vi "HFRR ADV v04.vi"() -> ()   [LabVIEW 2025] (continued)
                }
                frame 94 {
                  n2376 = local write "S 96"(w3499) -> ()
                }
                frame 95 {
                  n2377 = local write "S 97"(w3500) -> ()
                }
                frame 96 {
                  n2378 = local write "S 98"(w3501) -> ()
                }
                frame 97 {
                  n2379 = local write "S 99"(w3502) -> ()
                }
                frame 98 {
                  n2380 = local write "S 100"(w3503) -> ()
                }
                frame 99 {
                  n2381 = local write "S 101"(w3504) -> ()
                }
                frame 100 {
                  n2382 = local write "S 102"(w3505) -> ()
                }
                frame 101 {
                  n2383 = local write "S 103"(w3506) -> ()
                }
                frame 102 {
                  n2384 = local write "S 104"(w3507) -> ()
                }
                frame 103 {
                  n2385 = local write "S 105"(w3508) -> ()
                }
                frame 104 {
                  n2386 = local write "S 106"(w3509) -> ()
                }
                frame 105 {
                }
                frame 106 {
                  n2387 = property on="OK Button 17" class="Bool (strict)"("Boolean Text.Text"=w3510) -> ()  [unwired: 2 in, 2 out]
                }
                frame 107 {
                  n2388 = property on="OK Button 16" class="Bool (strict)"("Boolean Text.Text"=w3511) -> ()  [unwired: 2 in, 2 out]
                }
                frame 108 {
                  n2389 = property on="TITTLE" class="Str"("Caption.Text"=w3512) -> ()  [unwired: 2 in, 2 out]
                }
                frame 109 {
                  "String 30" <- w3513
                }
                frame 110 {
                  n2390 = property on="Test Date" class="Str"("Caption.Text"=w3514) -> ()  [unwired: 2 in, 2 out]
                  "String 31" <- w3514
                }
                frame 111 {
                  n2391 = property on="Sample ID" class="Str"("Caption.Text"=w3515) -> ()  [unwired: 2 in, 2 out]
                  "String 32" <- w3515
                }
                frame 112 {
                  n2392 = property on="Tested by" class="Str"("Caption.Text"=w3516) -> ()  [unwired: 2 in, 2 out]
                  "String 33" <- w3516
                }
                frame 113 {
                  n2393 = property on="System Configured Printers 2" class="Arr (strict)"("Caption.Text"=w3517) -> ()  [unwired: 2 in, 2 out]
                }
                frame 114 {
                  n2394 = property on="Selected Printer" class="Str"("Caption.Text"=w3518) -> ()  [unwired: 2 in, 2 out]
                }
                frame 115 {
                  n2395 = property on="Select Printer 3" class="DigNum (strict)"("Caption.Text"=w3519) -> ()  [unwired: 2 in, 2 out]
                }
                frame 116 {
                  n2396 = property on="Print" class="Bool (strict)"("Boolean Text.Text"=w3520) -> ()  [unwired: 2 in, 2 out]
                }
                frame 117 {
                  "String 41" <- w3521
                }
                frame 118 {
                  n2397 = property on="tested by" class="Str"("Caption.Text"=w3522) -> ()  [unwired: 2 in, 2 out]
                }
                frame 119 {
                }
                frame 120 {
                  n2398 = property on="Export" class="Bool (strict)"("Boolean Text.Text"=w3523) -> ()  [unwired: 2 in, 2 out]
                }
                frame 121 {
                  n2399 = property on="TEMP INTERCEPT:" class="DigNum (strict)"("Caption.Text"=w3524) -> ()  [unwired: 2 in, 2 out]
                }
                frame 122 {
                  n2400 = property on="AIR TEMP INTERCEPT:" class="DigNum (strict)"("Caption.Text"=w3525) -> ()  [unwired: 2 in, 2 out]
                }
                frame 123 {
                  n2401 = property on="Select File Type" class="Enum (strict)"("Caption.Text"=w3526) -> ()  [unwired: 2 in, 2 out]
                }
                frame 124 {
                  n2402 = property on="s.NO" class="Str"("Caption.Text"=w3527) -> ()  [unwired: 2 in, 2 out]
                  "String 45" <- w3527
                }
                frame 125 {
                  n2403 = property on="trip1 8" class="Bool (strict)"("Boolean Text.Text"=w3528) -> ()  [unwired: 2 in, 2 out]
                }
                frame 126, Default {
                }
              }
            }
          }
          frame #1 {
            w3536 = TRUE ("Visible")
            n2404 = local read "S 91"() -> (w3553:string)
            n2405 = local read "S 90"() -> (w3552:string)
            n2406 = local read "S 88"() -> (w3551:string)
            n2407 = property on="Threshold" class="DigNum (strict)"("Caption.Text"=w3553) -> ()  [unwired: 2 in, 2 out]
            n2408 = property on="File Path" class="Path"("Caption.Text"=w3552) -> ()  [unwired: 2 in, 2 out]
            n2409 = property on="SrvM CP" class="Bool (strict)"("Boolean Text.Text"=w3551) -> ()  [unwired: 2 in, 2 out]
            n2410 = local read "S 71"() -> (w3546:string)
            n2411 = local read "S 86"() -> (w3548:string)
            n2412 = local read "S 85"() -> (w3549:string)
            n2413 = local read "S 87"() -> (w3547:string)
            n2414 = local read "S 84"() -> (w3550:string)
            n2415 = local read "S 103"() -> (w3535:string)
            n2416 = local read "S 104"() -> (w3534:string)
            n2417 = property on="ENTER THE NEW PASSWORD" class="Str"("Caption.Text"=w3547) -> ()  [unwired: 2 in, 2 out]
            n2418 = property on="Password" class="Str"("Caption.Text"=w3549) -> ()  [unwired: 2 in, 2 out]
            n2419 = property on="ENTER CURRENT PASSWORD" class="Str"("Caption.Text"=w3548) -> ()  [unwired: 2 in, 2 out]
            n2420 = property on="EDIT" class="Bool (strict)"("Boolean Text.Text"=w3546) -> ()  [unwired: 2 in, 2 out]
            n2421 = property on="SAVE" class="Bool (strict)"("Boolean Text.Text"=w3550) -> ()  [unwired: 2 in, 2 out]
            n2422 = Build Array(w3535, w3534) -> (w3533:string[])
            n2423 = property on="Heater Button" class="Bool (strict)"("Strings [4]"=w3533) -> ()  [unwired: 2 in, 2 out]
            n2424 = property on="CH-HUMIDITY WET" class="DigNum (strict)"("Caption.Size to Text?"=w3536) -> ()  [unwired: 2 in, 2 out]
            n2425 = property on="CH-HUMIDITY DRY" class="DigNum (strict)"("Caption.Size to Text?"=w3536) -> ()  [unwired: 2 in, 2 out]
            n2426 = property on="CH-POWER -" class="DigNum (strict)"("Caption.Size to Text?"=w3536) -> ()  [unwired: 2 in, 2 out]
            n2427 = property on="CH-HEATER" class="DigNum (strict)"("Caption.Size to Text?"=w3536) -> ()  [unwired: 2 in, 2 out]
            n2428 = property on="CH-POWER +" class="DigNum (strict)"("Caption.Size to Text?"=w3536) -> ()  [unwired: 2 in, 2 out]
            n2429 = local read "S 92"() -> (w3545:string)
            n2430 = local read "S 93"() -> (w3544:string)
            n2431 = local read "S 105"() -> (w3531:string)
            n2432 = local read "S 106"() -> (w3530:string)
            n2433 = Build Array(w3545, w3544) -> ()  [unwired: 1 out]
            n2434 = Build Array(w3531, w3530) -> (w3532:string[])
            n2435 = local read "S 95"() -> (w3542:string)
            n2436 = local read "S 94"() -> (w3543:string)
            n2437 = local read "bs"() -> (w3558:string)
            n2438 = local read "as"() -> (w3559:string)
            n2439 = property on="Humidity" class="Bool (strict)"("Strings [4]"=w3532) -> ()  [unwired: 2 in, 2 out]
            n2440 = Concatenate Strings(w3558, "\r", w3559) -> ()  [unwired: 1 out]
            n2441 = property on="STROKE GAIN :" class="DigNum (strict)"("Caption.Text"=w3542) -> ()  [unwired: 2 in, 2 out]
            n2442 = property on="DISPLACEMENT :" class="DigNum (strict)"("Caption.Text"=w3543) -> ()  [unwired: 2 in, 2 out]
            n2443 = property on="Rh After" class="DigNum (strict)"("Caption.Size to Text?"=TRUE ("Caption.Size to Text")) -> ()  [unwired: 2 in, 2 out]
            n2444 = local read "S 48"() -> (w3582:string)
            n2445 = local read "S 50"() -> (w3580:string)
            n2446 = local read "S 51"() -> (w3579:string)
            n2447 = local read "S 49"() -> (w3581:string)
            n2448 = local read "S 52"() -> (w3578:string)
            n2449 = local read "as"() -> (w3563:string)
            n2450 = local read "bs"() -> (w3564:string)
            n2451 = local read "S 56"() -> (w3577:string)
            n2452 = local read "S 57"() -> (w3576:string)
            n2453 = local read "S 58"() -> (w3575:string)
            n2454 = local read "S 59"() -> (w3574:string)
            n2455 = property on="OPEN" class="Bool (strict)"("Boolean Text.Text"=w3578) -> ()  [unwired: 2 in, 2 out]
            n2456 = property on="OPEN 1" class="Bool (strict)"("Boolean Text.Text"=w3582) -> ()  [unwired: 2 in, 2 out]
            n2457 = property on="OPEN 2" class="Bool (strict)"("Boolean Text.Text"=w3581) -> ()  [unwired: 2 in, 2 out]
            n2458 = property on="OPEN 3" class="Bool (strict)"("Boolean Text.Text"=w3580) -> ()  [unwired: 2 in, 2 out]
            n2459 = property on="OPEN 4" class="Bool (strict)"("Boolean Text.Text"=w3579) -> ()  [unwired: 2 in, 2 out]
            n2460 = Concatenate Strings(w3564, "\r", w3563) -> ()  [unwired: 1 out]
            n2461 = local read "S 102"() -> (w3537:string)
            n2462 = property on="КОФ1" class="DigNum (strict)"("Caption.Text"=w3577) -> ()  [unwired: 2 in, 2 out]
            n2463 = local read "S 98"() -> (w3541:string)
            n2464 = local read "S 99"() -> (w3540:string)
            n2465 = local read "S 100"() -> (w3539:string)
            n2466 = local read "S 101"() -> (w3538:string)
            n2467 = property on="КОФ2" class="DigNum (strict)"("Caption.Text"=w3576) -> ()  [unwired: 2 in, 2 out]
            n2468 = property on="КОФ3" class="DigNum (strict)"("Caption.Text"=w3575) -> ()  [unwired: 2 in, 2 out]
            n2469 = property on="КОФ4" class="DigNum (strict)"("Caption.Text"=w3574) -> ()  [unwired: 2 in, 2 out]
            n2470 = local read "bs"() -> (w3562:string)
            n2471 = local read "as"() -> (w3561:string)
            n2472 = property on="CH-POWER +" class="DigNum (strict)"("Caption.Text"=w3541) -> ()  [unwired: 2 in, 2 out]
            n2473 = property on="CH-POWER -" class="DigNum (strict)"("Caption.Text"=w3540) -> ()  [unwired: 2 in, 2 out]
            n2474 = property on="CH-HEATER" class="DigNum (strict)"("Caption.Text"=w3539) -> ()  [unwired: 2 in, 2 out]
            n2475 = property on="CH-HUMIDITY DRY" class="DigNum (strict)"("Caption.Text"=w3538) -> ()  [unwired: 2 in, 2 out]
            n2476 = property on="CH-HUMIDITY WET" class="DigNum (strict)"("Caption.Text"=w3537) -> ()  [unwired: 2 in, 2 out]
            n2477 = local read "S 60"() -> (w3573:string)
            n2478 = local read "S 54"() -> (w3583:string)
            n2479 = Concatenate Strings(w3562, "\r", w3561) -> ()  [unwired: 1 out]
            n2480 = Concatenate Strings(w3583, w3573) -> ()  [unwired: 1 out]
            n2481 = local read "S 77"() -> (→"String 43":string)
            n2482 = local read "S 76"() -> (w3556:string)
            n2483 = local read "S 78"() -> (w3555:string)
            n2484 = local read "S 71"() -> (w3567:string)
            n2485 = local read "S 66"() -> (w3572:string)
            n2486 = local read "S 67"() -> (w3571:string)
            n2487 = local read "S 68"() -> (w3570:string)
            n2488 = local read "S 69"() -> (w3569:string)
            n2489 = local read "S 70"() -> (w3568:string)
            n2490 = property on="AIR TEMP" class="DigNum (strict)"("Caption.Text"=w3555) -> ()  [unwired: 2 in, 2 out]
            n2491 = property on="Set Strk" class="DigNum (strict)"("Caption.Text"=w3556) -> ()  [unwired: 2 in, 2 out]
            n2492 = property on="FRIC. FORCE :" class="DigNum (strict)"("Caption.Text"=w3572) -> ()  [unwired: 2 in, 2 out]
            n2493 = property on="TEMPERATURE :" class="DigNum (strict)"("Caption.Text"=w3571) -> ()  [unwired: 2 in, 2 out]
            n2494 = property on="SPEED OUT:" class="DigNum (strict)"("Caption.Text"=w3570) -> ()  [unwired: 2 in, 2 out]
            n2495 = property on="AIR TEMPERATURE :" class="DigNum (strict)"("Caption.Text"=w3569) -> ()  [unwired: 2 in, 2 out]
            n2496 = property on="HUMIDITY:" class="DigNum (strict)"("Caption.Text"=w3568) -> ()  [unwired: 2 in, 2 out]
            n2497 = property on="EDIT" class="Bool (strict)"("Boolean Text.Text"=w3567) -> ()  [unwired: 2 in, 2 out]
            n2498 = local read "S 79"() -> (w3554:string)
            n2499 = property on="Stroke" class="DigNum (strict)"("Caption.Text"=w3554) -> ()  [unwired: 2 in, 2 out]
          }
          frame #2 {
          }
        }
        n2500 = local write "Lan flag"(10.0 ("Lan flag")) -> ()
      }
      frame Enabled {
      }
    }
    n2501 = Wait (ms)(milliseconds to wait=u32 2000) -> ()  [unwired: 1 out]
    n2502 = local read "EXIT"() -> (w3359:bool)
  }
  n2503 = while {
    tunnel: [w3591] -> w37
    i -> [w3590]
    stop <- w3591 stop-if-true
    n2504 = local read "EXIT"() -> (w3591:bool)
    n2505 = Equal To 0?(x=w3590) -> (x = 0?=w3588:bool)
    n2506 = call "Elapsed Time3"("Time Target (s)"=45.0, "Auto Reset"=TRUE) -> ("Time has Elapsed"=w3587:bool)  [unwired: 10 in, 7 out]
    n2507 = Wait (ms)(milliseconds to wait=u32 50) -> ()  [unwired: 1 out]
    n2508 = Or(x=w3587, y=w3588) -> (x .or. y?=w3589:bool)
    n2509 = case shown="True" w3589 {
      frame False {
      }
      frame True {
        n2510 = call <vilib>:"System Exec.vi"("run minimized? (F)"=TRUE, "error in (no error)"="error in (no error)", "command line"="powercfg.exe -change -monitor-timeout-ac 0") -> ("error out"=w3602:errorcluster)  [unwired: 5 in, 3 out]
        n2511 = call <vilib>:"System Exec.vi"("run minimized? (F)"=TRUE, "error in (no error)"=w3602, "command line"="powercfg.exe -change -disk-timeout-ac 0") -> ("error out"=w3601:errorcluster)  [unwired: 5 in, 3 out]
        n2512 = call <vilib>:"System Exec.vi"("run minimized? (F)"=TRUE, "error in (no error)"=w3601, "command line"="powercfg.exe -change -standby-timeout-ac 0") -> ("error out"=w3600:errorcluster)  [unwired: 5 in, 3 out]
        n2513 = call <vilib>:"System Exec.vi"("run minimized? (F)"=TRUE, "error in (no error)"=w3600, "command line"="powercfg.exe -change -hibernate-timeout-ac 0") -> ("error out"=w3599:errorcluster)  [unwired: 5 in, 3 out]
        n2514 = call <vilib>:"Simple Error Handler.vi"("error in (no error)"=w3599) -> ("error out"=w3605:errorcluster)  [unwired: 4 in, 4 out]
        n2515 = call <vilib>:"Clear Errors.vi"("error in (no error)"=w3605) -> ("error out"=→"error out":errorcluster)  [unwired: 5 in, 1 out]
      }
    }
  }
  n2516 = Compound Arithmetic op=OR(w40, w41, w37) -> (w39:bool)
  n2517 = flat-sequence {
    tunnel: w39 -> [_]
    frame #0 {
    }
    frame #1 {
      n2518 = Quit LabVIEW(quit? (T)=TRUE) -> ()
      n2519 = local write "EXIT"(FALSE ("EXIT")) -> ()
    }
  }
  n2520 = property on="Heater Button" class="Bool (strict)"("Visible"=TRUE) -> ()  [unwired: 2 in, 2 out]
  n2521 = while {
    shift-right: [w3614] -> _
    shift-left: _ -> [w3615]
    shift-right: [w3612] -> _
    shift-left: T13 {"Read Heave and Surge"="", "Bytes at Heave Port"=0.0, "Heave and Surge COM Port:"="COM9", "Com Port 2"="COM7", "Residual Due"="", "Heave COM Status 2"=TRUE, "Heave COM Status"=TRUE, "Port 2"=TRUE, "Sway PPR"=6400.0, "Surge PPR"=6400.0, "Heave PPR"=6400.0, "Sway Pitch"=2.0, "Surge Pitch"=3.0, "Heave Pitch"=4.0, "Sway Pulses/mm"=320.0, "Surge Pulses/mm"=1600.0, "Heave Pulses/mm"=1600.0, "inner loop"=0.0, "Read Heave and Surge 2"="", "String 36"="", "Write S"=FALSE, "WriteCC1"=[""], "Heave COM Loop"=0, "LastCom"="", "EXIT"=FALSE, "Error Heave"={"status"=TRUE, "code"=-1073807343, "source"=""}} -> [w3611]
    shift-right: [w3609] -> _
    shift-left: enum16{"init", "MAIN", "Panel Close"}."init" -> [w3610]
    stop <- w3613 stop-if-true
    n2522 = case shown="\"MAIN\"" w3610 {
      tunnel: w3615 -> [w3629 w3644 w3714 w3716]
      tunnel: [w3623 w3662 w3714 w3716] -> w3614
      tunnel: [_ _ TRUE _] -> w3613
      tunnel: [w3619 w3659 w3712 w3715] -> w3612
      tunnel: w3611 -> [w3626 w3643 w3712 w3715]
      tunnel: [enum16{"init", "MAIN", "Panel Close"}."MAIN" w3637 _ _] -> w3609
      frame "init" {
        n2523 = Bundle By Name(cluster=w3626, "Heave and Surge COM Port:"="Instrument Com Port") -> (w3625:T13)
        n2524 = call "Instrument fgv.vi"("Enum"=T21."INIT", "error in (no error) 2"=w3629, "INPUT"=w3625) -> ("error"=w3627:errorcluster, "output"=w3622:T13)  [unwired: 6 in, 1 out]
        n2525 = case shown="Error" w3627 {
          selector: w3627 -> [w3631 _]
          tunnel: [w3631 w3635] -> w3623
          tunnel: w3622 -> [w3630 w3633]
          tunnel: [w3630 w3632] -> w3620
          frame No Error {
          }
          frame Error {
            n2526 = call "Instrument fgv.vi"("Enum"=T21."ERROR INIT", "INPUT"=w3633) -> ("error"=w3636:errorcluster, "output"=w3632:T13)  [unwired: 7 in, 1 out]
            n2527 = call <vilib>:"Clear Errors.vi"("error in (no error)"=w3636) -> ("error out"=w3635:errorcluster)  [unwired: 5 in, 1 out]
          }
        }
        n2528 = local read "LastCom"() -> (w3618:string)
        n2529 = Unbundle By Name(w3620) -> ("Heave COM Status 2"=→"Heave COM Status 2" →"Instrument Status":bool, "Error Heave"=→"Error Heave":errorcluster)  [unwired: 1 out]
        n2530 = Bundle By Name(cluster=w3620, "LastCom"=w3618) -> (w3619:T13)
      }
      frame "MAIN" {
        n2531 = Unbundle By Name(w3643) -> ("Com Port 2"=w3664:refnum<visa-resource-name>)
        n2532 = local read "Instrument Com Port"() -> (w3641:refnum<visa-resource-name>)
        n2533 = local write "Com Port 4"(w3664) -> ()
        n2534 = Divide(x="Heave PPR", y="Heave Pitch") -> (x/y=→"Heave Pulses/mm":dbl)
        n2535 = Bundle By Name(cluster=w3643, "Heave and Surge COM Port:"=w3641) -> (w3642:T13)
        n2536 = Equal?(x=w3664, y=w3641) -> (x = y?=w3663:bool)
        n2537 = Divide(x="Sway PPR", y="Sway Pitch") -> (x/y=→"Sway Pulses/mm":dbl)
        n2538 = case shown="True" w3663 {
          tunnel: [w3668 w3685] -> w3662
          tunnel: w3644 -> [w3669 w3691]
          tunnel: w3642 -> [w3667 w3689]
          tunnel: [w3666 w3684] -> w3659
          frame False {
            n2539 = call <vilib>:"Clear Errors.vi"("error in (no error)"=w3669) -> ("error out"=w3665:errorcluster)  [unwired: 5 in, 1 out]
            n2540 = call "Instrument fgv.vi"("Enum"=T21."ERROR INIT", "error in (no error) 2"=w3665, "INPUT"=w3667) -> ("error"=w3671:errorcluster, "output"=w3666:T13)  [unwired: 6 in, 1 out]
            n2541 = call <vilib>:"Clear Errors.vi"("error in (no error)"=w3671) -> ("error out"=w3668:errorcluster)  [unwired: 5 in, 1 out]
          }
          frame True {
            n2542 = call "Instrument fgv.vi"("Enum"=T21."READ", "error in (no error) 2"=w3691, "INPUT"=w3689) -> ("error"=w3690:errorcluster, "output"=w3681:T13)  [unwired: 6 in, 1 out]
            n2543 = Bundle By Name(cluster=w3681, "String 36"="String") -> (w3680:T13)
            n2544 = case shown="True" "Write S" {
              selector: "Write S" -> [_ w3711]
              tunnel: w3690 -> [w3704 w3710]
              tunnel: [w3704 w3709] -> w3677
              tunnel: w3680 -> [w3703 w3706]
              tunnel: [w3703 w3705] -> w3676
              frame False {
              }
              frame True {
                n2545 = Not(x=w3711) -> (.not. x?=w3707:bool)
                n2546 = local write "Write S"(w3707) -> ()
                n2547 = call "Instrument fgv.vi"("Enum"=T21."MANUAL WRITE", "error in (no error) 2"=w3710, "INPUT"=w3706) -> ("error"=w3709:errorcluster, "output"=w3705:T13)  [unwired: 6 in, 1 out]
              }
            }
            n2548 = Array Size(array="WriteCC1") -> (size(s)=w3674:i32)
            n2549 = Greater Than 0?(x=w3674) -> (x > 0?=w3672:bool)
            n2550 = call "Instrument fgv.vi"("Enum"=T21."WRITE", "error in (no error) 2"=w3677, "WriteCC1"="WriteCC1", "INPUT"=w3676) -> ("error"=w3687:errorcluster, "WriteCC1 2"=w3675:string[], "output"=w3686:T13)  [unwired: 5 in]
            n2551 = case shown="True" w3672 {
              tunnel: w3675 -> [_ w3693]
              frame False {
              }
              frame True {
                n2552 = local write "WriteCC1"(w3693) -> ()
              }
            }
            n2553 = case shown="Error" w3687 {
              selector: w3687 -> [w3694 w3697]
              tunnel: w3686 -> [w3695 w3702]
              tunnel: [w3695 w3701] -> w3684
              tunnel: [w3694 w3699] -> w3685
              frame No Error {
              }
              frame Error {
                n2554 = call <vilib>:"Clear Errors.vi"("error in (no error)"=w3697) -> ("error out"=w3696:errorcluster)  [unwired: 5 in, 1 out]
                n2555 = call "Instrument fgv.vi"("Enum"=T21."ERROR INIT", "error in (no error) 2"=w3696, "INPUT"=w3702) -> ("error"=w3700:errorcluster, "output"=w3701:T13)  [unwired: 6 in, 1 out]
                n2556 = call <vilib>:"Clear Errors.vi"("error in (no error)"=w3700) -> ("error out"=w3699:errorcluster)  [unwired: 5 in, 1 out]
              }
            }
            n2557 = Unbundle By Name(w3684) -> ("LastCom"=→"LastCom":string, "Read Heave and Surge"=→"Read Humidity":string)
          }
        }
        n2558 = Divide(x="Surge PPR", y="Surge Pitch") -> (x/y=→"Surge Pulses/mm":dbl)
        n2559 = Unbundle By Name(w3659) -> ("Heave COM Status 2"=w3661:bool, "Heave COM Status"=w3660:bool, "Error Heave"=w3657:errorcluster, "Bytes at Heave Port"=→"Bytes at Humidity Port":dbl)
        n2560 = Unbundle By Name(w3657) -> ("status"=→"Port 5":bool)
        n2561 = local write "Error Heave"(w3657) -> ()
        n2562 = Not(x=w3660) -> (.not. x?=w3645:bool)
        n2563 = Not(x=w3661) -> (.not. x?=w3646:bool)
        n2564 = local write "Instrument Status"(w3645) -> ()
        n2565 = local write "Heave COM Status 2"(w3646) -> ()
        n2566 = local read "Quit"() -> (w3638:bool)
        n2567 = Select(t=enum16{"init", "MAIN", "Panel Close"}."Panel Close", s=w3638, f=enum16{"init", "MAIN", "Panel Close"}."MAIN") -> (s? t:f=w3637:enum16{"init", "MAIN", "Panel Close"})
      }
      frame "Panel Close" {
      }
      frame Default {
      }
    }
  }
  n2568 = while {
    stop <- w3738 stop-if-true
    n2569 = local read "Read Humidity"() -> (w3734:string)
    n2570 = call <vilib>:"High Resolution Polling Wait.vi"("seconds to wait"=0.1) -> ()  [unwired: 10 in, 1 out]
    n2571 = Spreadsheet String To Array(delimiter (Tab)=",", format string="", spreadsheet string=w3734, array type (2D Dbl)=string[] []) -> (array=w3732:string[])
    n2572 = for {
      tunnel: w3732 -> [w3741] mode=indexing
      tunnel: string[] ["STATE;", "SET;", "RH;", "T;", "AMB_RH;", "AMB_T;", "PUMP;", "FAN_IN;", "FAN_OUT;", "DEHUM;", "CURRENT;", "STALL;"] -> [w3740] mode=indexing
      tunnel: [w3739] -> w3731 mode=indexing
      n2573 = Match Pattern(string=w3741, regular expression=w3740) -> (after substring=w3739:string)  [unwired: 1 in, 3 out]
    }
    n2574 = Index Array(array=w3731) -> (element #1=→"STATE :":string, element #2=→"SET :":string, element #3=w3719:string, element #4=w3718:string, element #5=→"AMB_RH :":string, element #6=→"AMB_T :":string, element #7=→"PUMP :":string, element #8=→"FAN_IN :":string, element #9=→"FAN_OUT :":string, element #10=→"DEHUM :":string, element #11=→"CURRENT :":string, element #12=→"STALL :":string)  [unwired: 12 in]
    "RH :" <- w3719
    "T :" <- w3718
    n2575 = Fract/Exp String To Number(string=w3719) -> (number=→"RH Numeric:":dbl)  [unwired: 3 in, 1 out]
    n2576 = Fract/Exp String To Number(string=w3718) -> ()  [unwired: 3 in, 2 out]
    n2577 = local read "Quit"() -> (w3738:bool)
  }
  n2578 = disable-structure shown="Disabled" {
    disable-tunnel: w15 -> [w3742 _]
    frame Disabled {
      n2579 = while {
        tunnel: w3742 -> [_]
        tunnel: [w3743] -> _
        i -> [w3743]
        stop <- w3744 continue-if-true
        n2580 = Wait (ms)(milliseconds to wait=u32 50) -> ()  [unwired: 1 out]
        n2581 = stacked-sequence {
          frame #0 {
            # "Controls Text color"
            # "Controls BG color"
            n2582 = property on="FILE" class="Str"("Text.Text Colors:Text Color"="SC  Text") -> ()  [unwired: 2 in, 2 out]
            n2583 = property on="Fuel Discription :" class="Str"("Text.Text Colors:Text Color"="SC  Text") -> ()  [unwired: 2 in, 2 out]
            n2584 = property on="tested by" class="Str"("Text.Text Colors:Text Color"="SC  Text") -> ()  [unwired: 2 in, 2 out]
            n2585 = property on="Remarks :" class="Str"("Text.Text Colors:Text Color"="SC  Text") -> ()  [unwired: 2 in, 2 out]
            n2586 = property class="DigNum (strict)"("Numeric Text.Text Colors:BG Color"="NC BG") -> ()  [unwired: 2 in, 2 out]
            n2587 = property class="DigNum (strict)"("Numeric Text.Text Colors:BG Color"="NC BG") -> ()  [unwired: 2 in, 2 out]
            n2588 = property class="DigNum (strict)"("Numeric Text.Text Colors:BG Color"="NC BG") -> ()  [unwired: 2 in, 2 out]
            n2589 = property class="DigNum (strict)"("Numeric Text.Text Colors:BG Color"="NC BG") -> ()  [unwired: 2 in, 2 out]
            n2590 = property class="DigNum (strict)"("Numeric Text.Text Colors:BG Color"="NC BG") -> ()  [unwired: 2 in, 2 out]
            n2591 = property class="DigNum (strict)"("Numeric Text.Text Colors:BG Color"="NC BG") -> ()  [unwired: 2 in, 2 out]
            n2592 = property class="DigNum (strict)"("Numeric Text.Text Colors:BG Color"="NC BG") -> ()  [unwired: 2 in, 2 out]
            n2593 = property class="DigNum (strict)"("Numeric Text.Text Colors:BG Color"="NC BG") -> ()  [unwired: 2 in, 2 out]
            n2594 = property class="DigNum (strict)"("Numeric Text.Text Colors:BG Color"="NC BG") -> ()  [unwired: 2 in, 2 out]
            n2595 = property class="DigNum (strict)"("Numeric Text.Text Colors:BG Color"="NC BG") -> ()  [unwired: 2 in, 2 out]
            n2596 = property class="DigNum (strict)"("Numeric Text.Text Colors:BG Color"="NC BG") -> ()  [unwired: 2 in, 2 out]
            n2597 = property class="DigNum (strict)"("Numeric Text.Text Colors:BG Color"="NC BG") -> ()  [unwired: 2 in, 2 out]
            n2598 = property on="FILE" class="Str"("Text.Text Colors:BG Color"="SC BG 3") -> ()  [unwired: 2 in, 2 out]
            n2599 = property on="Fuel Discription :" class="Str"("Text.Text Colors:BG Color"="SC BG 3") -> ()  [unwired: 2 in, 2 out]
            n2600 = property on="tested by" class="Str"("Text.Text Colors:BG Color"="SC BG 3") -> ()  [unwired: 2 in, 2 out]
            n2601 = property on="Remarks :" class="Str"("Text.Text Colors:BG Color"="SC BG 3") -> ()  [unwired: 2 in, 2 out]
            n2602 = property class="DigNum (strict)"("Numeric Text.Text Colors:Text Color"="NC Text") -> ()  [unwired: 2 in, 2 out]
            n2603 = property class="DigNum (strict)"("Numeric Text.Text Colors:Text Color"="NC Text") -> ()  [unwired: 2 in, 2 out]
            n2604 = property class="DigNum (strict)"("Numeric Text.Text Colors:Text Color"="NC Text") -> ()  [unwired: 2 in, 2 out]
            n2605 = property class="DigNum (strict)"("Numeric Text.Text Colors:Text Color"="NC Text") -> ()  [unwired: 2 in, 2 out]
            n2606 = property class="DigNum (strict)"("Numeric Text.Text Colors:Text Color"="NC Text") -> ()  [unwired: 2 in, 2 out]
            n2607 = property class="DigNum (strict)"("Numeric Text.Text Colors:Text Color"="NC Text") -> ()  [unwired: 2 in, 2 out]
            n2608 = property class="DigNum (strict)"("Numeric Text.Text Colors:Text Color"="NC Text") -> ()  [unwired: 2 in, 2 out]
            n2609 = property class="DigNum (strict)"("Numeric Text.Text Colors:Text Color"="NC Text") -> ()  [unwired: 2 in, 2 out]
            n2610 = property class="DigNum (strict)"("Numeric Text.Text Colors:Text Color"="NC Text") -> ()  [unwired: 2 in, 2 out]
            n2611 = property class="DigNum (strict)"("Numeric Text.Text Colors:Text Color"="NC Text") -> ()  [unwired: 2 in, 2 out]
            n2612 = property class="DigNum (strict)"("Numeric Text.Text Colors:Text Color"="NC Text") -> ()  [unwired: 2 in, 2 out]
            n2613 = property class="DigNum (strict)"("Numeric Text.Text Colors:Text Color"="NC Text") -> ()  [unwired: 2 in, 2 out]
            n2614 = property class="DigNum (strict)"("Numeric Text.Text Colors:Text Color"="NI Text  2") -> ()  [unwired: 2 in, 2 out]
            n2615 = property class="DigNum (strict)"("Numeric Text.Text Colors:Text Color"="NI Text  2") -> ()  [unwired: 2 in, 2 out]
            n2616 = property class="DigNum (strict)"("Numeric Text.Text Colors:Text Color"="NI Text  2") -> ()  [unwired: 2 in, 2 out]
            n2617 = property class="DigNum (strict)"("Numeric Text.Text Colors:Text Color"="NI Text  2") -> ()  [unwired: 2 in, 2 out]
            n2618 = property class="DigNum (strict)"("Numeric Text.Text Colors:Text Color"="NI Text  2") -> ()  [unwired: 2 in, 2 out]
            n2619 = property class="DigNum (strict)"("Numeric Text.Text Colors:Text Color"="NI Text  2") -> ()  [unwired: 2 in, 2 out]
            n2620 = property class="DigNum (strict)"("Numeric Text.Text Colors:Text Color"="NI Text  2") -> ()  [unwired: 2 in, 2 out]
            n2621 = property class="DigNum (strict)"("Numeric Text.Text Colors:Text Color"="NI Text  2") -> ()  [unwired: 2 in, 2 out]
            n2622 = property class="DigNum (strict)"("Numeric Text.Text Colors:Text Color"="NI Text  2") -> ()  [unwired: 2 in, 2 out]
            n2623 = property class="DigNum (strict)"("Numeric Text.Text Colors:Text Color"="NI Text  2") -> ()  [unwired: 2 in, 2 out]
            n2624 = property class="DigNum (strict)"("Numeric Text.Text Colors:Text Color"="NI Text  2") -> ()  [unwired: 2 in, 2 out]
            n2625 = property class="DigNum (strict)"("Numeric Text.Text Colors:Text Color"="NI Text  2") -> ()  [unwired: 2 in, 2 out]
            n2626 = property class="DigNum (strict)"("Numeric Text.Text Colors:Text Color"="NI Text  2") -> ()  [unwired: 2 in, 2 out]
            n2627 = property class="DigNum (strict)"("Numeric Text.Text Colors:Text Color"="NI Text  2") -> ()  [unwired: 2 in, 2 out]
            n2628 = property class="DigNum (strict)"("Numeric Text.Text Colors:Text Color"="NI Text  2") -> ()  [unwired: 2 in, 2 out]
            n2629 = property class="DigNum (strict)"("Numeric Text.Text Colors:Text Color"="NI Text  2") -> ()  [unwired: 2 in, 2 out]
            n2630 = property on="Coefficient Of Friction" class="XYGraph (strict)"("Plot Area:Colors:FG Color"="GFG  2", "Plot Area:Colors:BG Color"="GBG   2") -> ()  [unwired: 2 in, 2 out]
            n2631 = property on="Humidity" class="XYGraph (strict)"("Plot Area:Colors:FG Color"="GFG  2", "Plot Area:Colors:BG Color"="GBG   2") -> ()  [unwired: 2 in, 2 out]
            n2632 = property on="Air Temperature" class="XYGraph (strict)"("Plot Area:Colors:FG Color"="GFG  2", "Plot Area:Colors:BG Color"="GBG   2") -> ()  [unwired: 2 in, 2 out]
            n2633 = property on="Sample Temperature" class="XYGraph (strict)"("Plot Area:Colors:FG Color"="GFG  2", "Plot Area:Colors:BG Color"="GBG   2") -> ()  [unwired: 2 in, 2 out]
            n2634 = property class="DigNum (strict)"("Numeric Text.Text Colors:BG Color"="NI BG 2") -> ()  [unwired: 2 in, 2 out]
            n2635 = property class="DigNum (strict)"("Numeric Text.Text Colors:BG Color"="NI BG 2") -> ()  [unwired: 2 in, 2 out]
            n2636 = property class="DigNum (strict)"("Numeric Text.Text Colors:BG Color"="NI BG 2") -> ()  [unwired: 2 in, 2 out]
            n2637 = property class="DigNum (strict)"("Numeric Text.Text Colors:BG Color"="NI BG 2") -> ()  [unwired: 2 in, 2 out]
            n2638 = property class="DigNum (strict)"("Numeric Text.Text Colors:BG Color"="NI BG 2") -> ()  [unwired: 2 in, 2 out]
            n2639 = property class="DigNum (strict)"("Numeric Text.Text Colors:BG Color"="NI BG 2") -> ()  [unwired: 2 in, 2 out]
            n2640 = property class="DigNum (strict)"("Numeric Text.Text Colors:BG Color"="NI BG 2") -> ()  [unwired: 2 in, 2 out]
            n2641 = property class="DigNum (strict)"("Numeric Text.Text Colors:BG Color"="NI BG 2") -> ()  [unwired: 2 in, 2 out]
            n2642 = property class="DigNum (strict)"("Numeric Text.Text Colors:BG Color"="NI BG 2") -> ()  [unwired: 2 in, 2 out]
            n2643 = property class="DigNum (strict)"("Numeric Text.Text Colors:BG Color"="NI BG 2") -> ()  [unwired: 2 in, 2 out]
            n2644 = property class="DigNum (strict)"("Numeric Text.Text Colors:BG Color"="NI BG 2") -> ()  [unwired: 2 in, 2 out]
            n2645 = property class="DigNum (strict)"("Numeric Text.Text Colors:BG Color"="NI BG 2") -> ()  [unwired: 2 in, 2 out]
            n2646 = property class="DigNum (strict)"("Numeric Text.Text Colors:BG Color"="NI BG 2") -> ()  [unwired: 2 in, 2 out]
            n2647 = property class="DigNum (strict)"("Numeric Text.Text Colors:BG Color"="NI BG 2") -> ()  [unwired: 2 in, 2 out]
            n2648 = property class="DigNum (strict)"("Numeric Text.Text Colors:BG Color"="NI BG 2") -> ()  [unwired: 2 in, 2 out]
            n2649 = property class="DigNum (strict)"("Numeric Text.Text Colors:BG Color"="NI BG 2") -> ()  [unwired: 2 in, 2 out]
            n2650 = property class="Bool"("Colors [4]"="Boolean BC T & BG") -> ()  [unwired: 2 in, 2 out]
            n2651 = property on="Save & Continue" class="Bool (strict)"("Colors [4]"="Boolean BC T & BG") -> ()  [unwired: 2 in, 2 out]
            n2652 = property on="STOP 3" class="Bool (strict)"("Colors [4]"="Boolean BC T & BG") -> ()  [unwired: 2 in, 2 out]
            n2653 = property on="Heater Button" class="Bool (strict)"("Colors [4]"="Boolean BC T & BG") -> ()  [unwired: 2 in, 2 out]
            n2654 = property class="Bool"("Colors [4]"="Boolean BC T & BG") -> ()  [unwired: 2 in, 2 out]
            n2655 = property on="Humidity" class="Bool (strict)"("Colors [4]"="Boolean BC T & BG") -> ()  [unwired: 2 in, 2 out]
            n2656 = property class="Bool (strict)"("Colors [4]"="Boolean BC T & BG") -> ()  [unwired: 2 in, 2 out]
            n2657 = property on="RUN" class="Bool (strict)"("Colors [4]"="Boolean BC T & BG") -> ()  [unwired: 2 in, 2 out]
            n2658 = property on="trip1 8" class="Bool (strict)"("Colors [4]"="Boolean BC T & BG") -> ()  [unwired: 2 in, 2 out]
            n2659 = property class="Bool"("Colors [4]"="Boolean BC T & BG") -> ()  [unwired: 2 in, 2 out]
            n2660 = property class="Bool (strict)"("Colors [4]"="Boolean BC T & BG") -> ()  [unwired: 2 in, 2 out]
            n2661 = property on="OPEN 1" class="Bool (strict)"("Colors [4]"="Boolean BC T & BG 2") -> ()  [unwired: 2 in, 2 out]
            n2662 = property on="OPEN 2" class="Bool (strict)"("Colors [4]"="Boolean BC T & BG 2") -> ()  [unwired: 2 in, 2 out]
            n2663 = property on="OPEN 3" class="Bool (strict)"("Colors [4]"="Boolean BC T & BG 2") -> ()  [unwired: 2 in, 2 out]
            n2664 = property on="OPEN 4" class="Bool (strict)"("Colors [4]"="Boolean BC T & BG 2") -> ()  [unwired: 2 in, 2 out]
            n2665 = property on="OPEN" class="Bool (strict)"("Colors [4]"="Boolean BC T & BG 2") -> ()  [unwired: 2 in, 2 out]
            n2666 = property on="rstv2" class="Bool"("Colors [4]"="Boolean BC T & BG 2") -> ()  [unwired: 2 in, 2 out]
            n2667 = property on="RST CP" class="Bool"("Colors [4]"="Boolean BC T & BG 2") -> ()  [unwired: 2 in, 2 out]
            n2668 = property on="RSTV1 3" class="Bool"("Colors [4]"="Boolean BC T & BG 2") -> ()  [unwired: 2 in, 2 out]
            n2669 = property on="RSTV1 2" class="Bool"("Colors [4]"="Boolean BC T & BG 2") -> ()  [unwired: 2 in, 2 out]
          }
          frame #1 {
          }
        }
        n2670 = local read "EXIT"() -> (w3744:bool)
      }
    }
    frame Enabled {
    }
  }
  n2671 = disable-structure shown="Disabled" {
    frame Disabled {
      n2672 = while {
        tunnel: [w3989] -> _
        i -> [w3989]
        stop <- w3987 stop-if-true
        n2673 = local read "powstat"() -> (w3986:bool)
        n2674 = case shown="True" w3986 {
          frame False {
          }
          frame True {
            n2675 = local read "RUN"() -> (w3990:bool)
            n2676 = case shown="True" w3990 {
              frame False {
                w4020 = 65.0 ("y")
                n2677 = local read "Set Hz"() -> (w4048:dbl)
                n2678 = local read "NORMAL LOAD"() -> (w4049:dbl)
                n2679 = Multiply(x=w4048, y=60.0) -> (x*y=w4055:dbl)
                n2680 = Multiply(x=1.2 ("y"), y=0.949) -> (x*y=w4024:dbl)
                n2681 = Multiply(x=1.2 ("y"), y=0.8166) -> (x*y=w4028:dbl)
                n2682 = Multiply(x=1.2 ("y"), y=0.851) -> (x*y=w4023:dbl)
                n2683 = local read "FF 2"() -> (w4047:dbl)
                n2684 = Absolute Value(x=w4055) -> (abs(x)=w4053:dbl)
                n2685 = local read "Stroke"() -> (w4022:dbl)
                n2686 = Less?(x=w4022, y=w4028) -> (x < y?=w4025:bool)
                n2687 = In Range and Coerce(upper limit=w4024, x=w4022, lower limit=w4023) -> (In Range?=w4026:bool)  [unwired: 1 out]
                n2688 = case shown="13.." w4047 {
                  tunnel: [1 2 3] -> w4045
                  frame 0..10, Default {
                    # "Normal"
                  }
                  frame 11, 12 {
                  }
                  frame 13.. {
                  }
                }
                "FF STATE" <- w4045
                n2689 = local read "TEMP"() -> (w4008:dbl)
                n2690 = case shown="3601.." w4053 {
                  tunnel: [1 2 3] -> w4051
                  frame 0..3000, Default {
                    # "Normal"
                  }
                  frame 3001..3600 {
                  }
                  frame 3601.. {
                  }
                }
                n2691 = case shown="11.." w4049 {
                  tunnel: [1 3] -> w4050
                  frame 1..10, Default {
                  }
                  frame 11.. {
                  }
                }
                "NL STATE" <- w4050
                n2692 = Multiply(x=1.2 ("y"), y=0.95) -> (x*y=w4038:dbl)
                n2693 = Multiply(x=w4020, y=0.954) -> (x*y=w4012:dbl)
                n2694 = Or(x=w4025, y=w4026) -> (x .or. y?=w4027:bool)
                n2695 = Greater Or Equal?(x=w4022, y=w4038) -> (x >= y?=w4035:bool)
                n2696 = Multiply(x=w4020, y=0.99) -> (x*y=w4009:dbl)
                n2697 = Greater Or Equal?(x=w4008, y=w4009) -> (x >= y?=w4014:bool)
                n2698 = Greater Or Equal?(x=w4008, y=w4012) -> (x >= y?=w4011:bool)
                n2699 = case shown="0, 1, Default" w4022 {
                  tunnel: [1 3] -> w4039
                  frame 0, 1, Default {
                  }
                  frame 2.. {
                  }
                }
                n2700 = case shown="True" w4035 {
                  tunnel: [1 3] -> w4040
                  frame False {
                  }
                  frame True {
                  }
                }
                n2701 = case shown="True" w4027 {
                  tunnel: [1 2] -> w4041
                  frame False {
                  }
                  frame True {
                  }
                }
                n2702 = case shown="..0" w4008 {
                  tunnel: [2 3 3 1] -> w4015
                  frame 61, 62 {
                  }
                  frame 63.. {
                  }
                  frame ..0 {
                  }
                  frame 10..60, Default {
                  }
                }
                n2703 = case shown="True" w4014 {
                  tunnel: [1 3] -> w4016
                  frame False {
                  }
                  frame True {
                  }
                }
                n2704 = Number To Decimal String(number=w4051) -> (decimal integer string=w4052:string)  [unwired: 1 in]
                n2705 = case shown="True" w4011 {
                  tunnel: [1 2] -> w4017
                  frame False {
                  }
                  frame True {
                  }
                }
                n2706 = Number To Decimal String(number=1) -> (decimal integer string=→"Air temp":string)  [unwired: 1 in]
                n2707 = Number To Decimal String(number=w4045) -> (decimal integer string=→"ff_st":string)  [unwired: 1 in]
                n2708 = local write "sp_st"(w4052) -> ()
                n2709 = Number To Decimal String(number=w4050) -> (decimal integer string=→"nl_st":string)  [unwired: 1 in]
                n2710 = Build Array(w4015, w4016, w4017) -> (w4018:i32[])
                n2711 = Build Array(w4039, w4040, w4041) -> (w4042:i32[])
                n2712 = Array Max & Min(array=w4018) -> (max value=w4019:i32)  [unwired: 3 out]
                n2713 = Array Max & Min(array=w4042) -> (max value=w4043:i32)  [unwired: 3 out]
                n2714 = Number To Decimal String(number=w4019) -> (decimal integer string=w4007:string)  [unwired: 1 in]
                n2715 = Number To Decimal String(number=w4043) -> (decimal integer string=→"Stroke Ln 2":string)  [unwired: 1 in]
                n2716 = local write "temp_st"(w4007) -> ()
              }
              frame True {
                w4105 = 65.0 ("y")
                # "Healthy -1\nWarning -2\nError -3"
                n2717 = local read "TEMP"() -> (w4116:dbl)
                n2718 = local read "NORMAL LOAD"() -> (w4120:dbl)
                n2719 = local read "Set Hz"() -> (w4118:dbl)
                n2720 = Multiply(x=1.2 ("y"), y=0.949) -> (x*y=w4100:dbl)
                n2721 = Multiply(x=1.2 ("y"), y=0.8166) -> (x*y=w4096:dbl)
                n2722 = Multiply(x=1.2 ("y"), y=0.851) -> (x*y=w4101:dbl)
                n2723 = Multiply(x=w4105, y=0.954) -> (x*y=w4112:dbl)
                n2724 = Multiply(x=w4105, y=0.99) -> (x*y=w4115:dbl)
                n2725 = Greater Or Equal?(x=w4116, y=w4115) -> (x >= y?=w4110:bool)
                n2726 = Multiply(x=w4118, y=60.0) -> (x*y=w4124:dbl)
                n2727 = Greater Or Equal?(x=w4116, y=w4112) -> (x >= y?=w4113:bool)
                n2728 = local read "FF 2"() -> (w4119:dbl)
                n2729 = local read "Stroke"() -> (w4102:dbl)
                n2730 = Less?(x=w4102, y=w4096) -> (x < y?=w4099:bool)
                n2731 = In Range and Coerce(upper limit=w4100, x=w4102, lower limit=w4101) -> (In Range?=w4098:bool)  [unwired: 1 out]
                n2732 = Absolute Value(x=w4124) -> (abs(x)=w4122:dbl)
                n2733 = case shown="63.." w4116 {
                  tunnel: [2 3 3 1] -> w4109
                  frame 61, 62 {
                  }
                  frame 63.. {
                  }
                  frame ..0 {
                  }
                  frame 10..60, Default {
                  }
                }
                n2734 = case shown="True" w4110 {
                  tunnel: [1 3] -> w4108
                  frame False {
                  }
                  frame True {
                  }
                }
                n2735 = case shown="True" w4113 {
                  tunnel: [1 2] -> w4107
                  frame False {
                  }
                  frame True {
                  }
                }
                n2736 = Multiply(x=1.2 ("y"), y=0.95) -> (x*y=w4086:dbl)
                n2737 = case shown="1..10, Default" w4120 {
                  tunnel: [1 3] -> w4127
                  frame 1..10, Default {
                  }
                  frame 11.. {
                  }
                }
                n2738 = case shown="0..10, Default" w4119 {
                  tunnel: [1 2 3] -> w4126
                  frame 0..10, Default {
                  }
                  frame 11, 12 {
                  }
                  frame 13.. {
                  }
                }
                n2739 = case shown="3601.." w4122 {
                  tunnel: [1 2 3] -> w4121
                  frame 0..3000, Default {
                    # "Normal"
                  }
                  frame 3001..3600 {
                  }
                  frame 3601.. {
                  }
                }
                n2740 = Or(x=w4099, y=w4098) -> (x .or. y?=w4097:bool)
                n2741 = Greater Or Equal?(x=w4102, y=w4086) -> (x >= y?=w4089:bool)
                n2742 = case shown="0, 1, Default" w4102 {
                  tunnel: [1 3] -> w4085
                  frame 0, 1, Default {
                  }
                  frame 2.. {
                  }
                }
                n2743 = case shown="True" w4089 {
                  tunnel: [1 3] -> w4084
                  frame False {
                  }
                  frame True {
                  }
                }
                n2744 = case shown="True" w4097 {
                  tunnel: [1 2] -> w4083
                  frame False {
                  }
                  frame True {
                  }
                }
                n2745 = Build Array(w4109, w4108, w4107) -> (w4106:i32[])
                n2746 = Number To Decimal String(number=w4121) -> (decimal integer string=→"sp_st":string)  [unwired: 1 in]
                n2747 = Array Max & Min(array=w4106) -> (max value=w4103:i32)  [unwired: 3 out]
                "TEMP STATE" <- w4103
                n2748 = Number To Decimal String(number=w4127) -> (decimal integer string=w4130:string)  [unwired: 1 in]
                n2749 = Number To Decimal String(number=w4126) -> (decimal integer string=w4128:string)  [unwired: 1 in]
                n2750 = Number To Decimal String(number=w4103) -> (decimal integer string=→"temp_st":string)  [unwired: 1 in]
                n2751 = Build Array(w4085, w4084, w4083) -> (w4082:i32[])
                n2752 = local write "nl_st"(w4130) -> ()
                n2753 = local write "ff_st"(w4128) -> ()
                n2754 = Number To Decimal String(number=1) -> (decimal integer string=w4125:string)  [unwired: 1 in]
                n2755 = Array Max & Min(array=w4082) -> (max value=w4081:i32)  [unwired: 3 out]
                n2756 = local write "Air temp"(w4125) -> ()
                n2757 = Number To Decimal String(number=w4081) -> (decimal integer string=w4080:string)  [unwired: 1 in]
                n2758 = local write "Stroke Ln 2"(w4080) -> ()
              }
            }
            n2759 = local read "Stroke Ln 2"() -> (w3992:string)
            n2760 = local read "nl_st"() -> (w3998:string)
            n2761 = local read "ff_st"() -> (w3995:string)
            n2762 = local read "sp_st"() -> (w3996:string)
            n2763 = local read "temp_st"() -> (w3997:string)
            n2764 = local read "Air temp"() -> (w3991:string)
            n2765 = Replace Array Subset(array="in", new element #1=w3998, index #1=1 ("index"), new element #2=w3995, index #2=2 ("index"), new element #3=w3997, index #3=3 ("index"), new element #4=w3996, index #4=4 ("index"), new element #5=w3992, index #5=5 ("index"), new element #6=w3991, index #6=6 ("index"), new element #7="Sensor State" ("new element/subarray"), index #7=0 ("index")) -> (→"out":string[])
          }
        }
        n2766 = Wait (ms)(milliseconds to wait=u32 10) -> ()  [unwired: 1 out]
        n2767 = local read "EXIT"() -> (w3987:bool)
      }
      n2768 = while {
        stop <- w3961 stop-if-true
        n2769 = local read "run replace"() -> (w3963:bool)
        n2770 = Wait (ms)(milliseconds to wait=u32 100) -> ()  [unwired: 1 out]
        n2771 = Equal?(x="FLAG 2", y=0.0) -> (x = y?=w3964:bool)
        n2772 = case shown="True" w3964 {
          frame False {
          }
          frame True {
            n2773 = local write "FLAG 2"(100.0 ("FLAG 2")) -> ()
            n2774 = call <vilib>:"Read Characters From File.vi"("file path (dialog if empty)"=path "C:/LAB-IQ-NXT/WO 2449 TT.sig", "convert eol? (no:F)"=FALSE ("append to file? (new file:F)")) -> ("character string"=w3967:string)  [unwired: 4 in, 3 out]
            n2775 = call <vilib>:"Read Characters From File.vi"("file path (dialog if empty)"=path "C:/LAB-IQ-NXT/WO 2449 TRH.sig", "convert eol? (no:F)"=FALSE ("append to file? (new file:F)")) -> ("character string"=w3968:string)  [unwired: 4 in, 3 out]
            n2776 = Decimal String To Number(string=w3967) -> (number=w3969:i32)  [unwired: 2 in, 1 out]
            n2777 = local write "Total No. of Tests"(w3969) -> ()
            n2778 = Decimal String To Number(string=w3968) -> (number=w3972:i32)  [unwired: 2 in, 1 out]
            n2779 = local write "SEN.RUN HRS"(w3972) -> ()
          }
        }
        n2780 = case shown="True" w3963 {
          frame False {
          }
          frame True {
            n2781 = Equal?(x="FLAG 4", y=0.0) -> (x = y?=w3976:bool)
            n2782 = case shown="False" w3976 {
              frame False {
                n2783 = Get Date/Time In Seconds() -> (seconds since 1Jan1904=w3982:timestamp)
                n2784 = local read "START 3"() -> (w3980:dbl)
                n2785 = To Double Precision Float(number=w3982) -> (double precision float=w3981:dbl)
                n2786 = Subtract(x=w3981, y=w3980) -> (x-y=→"SENSOR TIME":dbl)
              }
              frame True {
                n2787 = Get Date/Time In Seconds() -> (seconds since 1Jan1904=w3984:timestamp)
                n2788 = local write "FLAG 4"(100.0 ("FLAG")) -> ()
                n2789 = To Double Precision Float(number=w3984) -> (double precision float=→"START 3":dbl)
              }
            }
          }
        }
        n2790 = local read "EXIT"() -> (w3961:bool)
      }
      n2791 = while {
        shift-right: [w3761] -> _
        shift-left: _ -> [w3762]
        tunnel: [w3757] -> _
        i -> [w3757]
        stop <- w3756 stop-if-true
        n2792 = Wait (ms)(milliseconds to wait=u32 50 ("Refresh Rate (ms)")) -> ()  [unwired: 1 out]
        n2793 = local read "Json End Flg"() -> (w3758:bool)
        n2794 = Not(x="Upld AR 2") -> ()  [unwired: 1 out]
        n2795 = local read "Upld AR 2"() -> (w3759:bool)
        n2796 = call "Elapsed Time9"("Time Target (s)"="Sen.Upload Rate (s)", "Reset"=FALSE, "Auto Reset"=TRUE) -> ("Time has Elapsed"=w3768:bool)  [unwired: 9 in, 7 out]
        n2797 = Or(x=w3768, y=w3758) -> (x .or. y?=w3764:bool)
        n2798 = case shown="True" w3764 {
          frame False {
          }
          frame True {
            w3860 = "\"SensorName\":\"" ("string")
            w3830 = " \"},{"
            w3855 = "\",\"SensorState\":\""
            w3857 = "\",\"SensorModelNumber\":\"" ("string")
            w3856 = "\",\"SensorRuntimeHours\":\"" ("string")
            n2799 = local read "model num"() -> (w3854:string[])
            n2800 = local read "Sensor name"() -> (w3873:string[])
            n2801 = local read "run"() -> (w3844:string[])
            n2802 = local read "SENSOR TIME"() -> (w3800:dbl)
            n2803 = local read "out"() -> (w3793:string[])
            n2804 = local read "Total No. of Tests"() -> (w3798:dbl)
            n2805 = Select(t=60.0, s="Run test 3", f=3600.0) -> (s? t:f=w3808:dbl)
            n2806 = Index Array(array=w3854, index #1=1 ("index")) -> (element #1=w3853:string, element #2=w3852:string, element #3=w3851:string, element #4=w3850:string, element #5=w3849:string, element #6=w3848:string)  [unwired: 5 in]
            n2807 = Index Array(array=w3844, index #1=1 ("index")) -> (element #1=w3843:string, element #2=w3842:string, element #3=w3841:string, element #4=w3840:string, element #5=w3839:string, element #6=w3838:string)  [unwired: 5 in]
            n2808 = Index Array(array=w3873, index #1=1 ("index")) -> (element #1=w3872:string, element #2=w3871:string, element #3=w3870:string, element #4=w3869:string, element #5=w3859:string, element #6=w3858:string)  [unwired: 5 in]
            n2809 = Index Array(array=w3793, index #1=1 ("index")) -> (element #1=w3825:string, element #2=w3824:string, element #3=w3823:string, element #4=w3822:string, element #5=w3821:string, element #6=w3820:string)  [unwired: 5 in]
            n2810 = local read "SEN.RUN HRS"() -> (w3796:dbl)
            n2811 = Divide(x=w3800, y=w3808) -> (x/y=w3807:dbl)
            n2812 = Increment(x=w3807) -> (x+1=w3803:dbl)
            n2813 = Number To Decimal String(number=w3803) -> (decimal integer string=→"run hrs":string)  [unwired: 1 in]
            n2814 = Divide(x=w3796, y=3600.0 ("f")) -> (x/y=w3791:dbl)
            n2815 = Round To Nearest(number=w3791) -> (nearest integer value=w3789:dbl)
            n2816 = Number To Decimal String(number=w3789) -> (decimal integer string=w3790:string)  [unwired: 1 in]
            n2817 = Number To Decimal String(number=w3798) -> (decimal integer string=w3799:string)  [unwired: 1 in]
            n2818 = local read "Model No"() -> (w3804:string)
            n2819 = local read "UUID"() -> (w3899:string)
            n2820 = local read "Serial No"() -> (w3903:string)
            n2821 = local read "Secret Key"() -> (w3904:string)
            n2822 = Concatenate Strings("\",\"MachineSerialNumber\":\"" ("string"), w3903) -> (w3907:string)
            n2823 = Concatenate Strings("\",\"ModelNumber\":\"" ("string"), w3804) -> (w3805:string)
            n2824 = Concatenate Strings("\",\"MachineRuntimeHours\":\"" ("string"), w3790) -> (w3908:string)
            n2825 = Concatenate Strings("\",\"MachineRuntimeCycles\":\"", w3799) -> (w3901:string)
            n2826 = Concatenate Strings(w3857, w3853) -> (w3887:string)
            n2827 = Concatenate Strings(w3856, w3843) -> (w3888:string)
            n2828 = Concatenate Strings(w3855, w3825) -> (w3886:string)
            n2829 = Concatenate Strings(w3907, w3805, w3908, w3901) -> (w3910:string)
            n2830 = Concatenate Strings(w3857, w3852) -> (w3884:string)
            n2831 = Concatenate Strings(w3856, w3842) -> (w3883:string)
            n2832 = Concatenate Strings(w3855, w3824) -> (w3885:string)
            n2833 = Concatenate Strings(w3857, w3851) -> (w3879:string)
            n2834 = Concatenate Strings(w3856, w3841) -> (w3880:string)
            n2835 = Concatenate Strings(w3855, w3823) -> (w3878:string)
            n2836 = Concatenate Strings(w3857, w3850) -> (w3876:string)
            n2837 = Concatenate Strings(w3856, w3840) -> (w3875:string)
            n2838 = Concatenate Strings(w3855, w3822) -> (w3877:string)
            n2839 = Concatenate Strings(w3887, w3888, w3886) -> (w3889:string)
            n2840 = Concatenate Strings(w3857, w3849) -> (w3866:string)
            n2841 = Concatenate Strings(w3856, w3839) -> (w3867:string)
            n2842 = Concatenate Strings(w3857, w3848) -> (w3863:string)
            n2843 = Concatenate Strings(w3856, w3838) -> (w3862:string)
            n2844 = Concatenate Strings(w3855, w3821) -> (w3865:string)
            n2845 = Concatenate Strings(w3855, w3820) -> (w3864:string)
            n2846 = Concatenate Strings("{\"SecretKey\":\"", w3904, w3910, "\",\"UUID\" : \"", w3899, "\",\"SensorInformation\":", "[{" ("string")) -> (w3837:string)
            n2847 = Concatenate Strings(w3884, w3883, w3885) -> (w3882:string)
            n2848 = Concatenate Strings(w3879, w3880, w3878) -> (w3881:string)
            n2849 = Concatenate Strings(w3876, w3875, w3877) -> (w3874:string)
            n2850 = Concatenate Strings(w3866, w3867, w3865) -> (w3868:string)
